vi "Configure Auto Detect.vi"(6 "Manual Frequency (0 Hz)":i32, 7 "Frequency Source (0: tsMeasFreq)":i32(ring) items=["tsMeasFreq", "tsAnlgGenA", "tsAnlgGenB", "tsDigGenA", "tsDigGenB", "tsSweepSrc0", "tsSweepSrc1"], 8 "error in (no error)":errorcluster, 9 "Enable TDD Frequency Status (0: tmFixed)":i32(ring) items=["tmFixed", "tmTuned"], 10 "Analyzer (0: A0)":i32(ring) items=["A0", "A1"], 11 "VISA resource name":refnum<visa-resource-name>) -> (0 "error out":errorcluster, 3 "VISA resource name out":refnum<visa-resource-name>)   [LabVIEW 2014, in "Stanford Research SR1.lvlib"]
doc: "Configures the attributes for the Auto Detect."
uses:
  Stanford Research SR1.lvlib
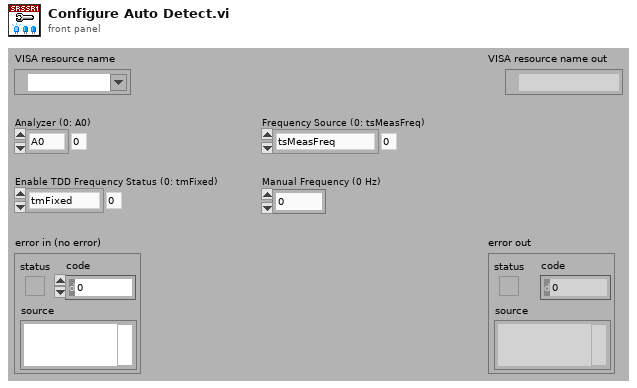
[diagram p1: front panel]
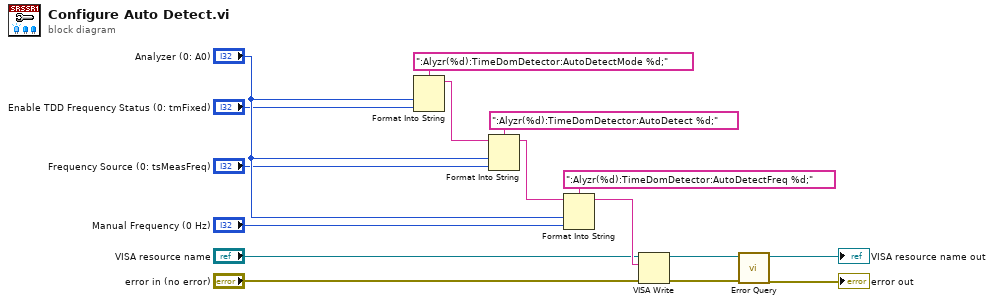
[diagram p0: block diagram]
diagram:
  n1 = Format Into String(format string=":Alyzr(%d):TimeDomDetector:AutoDetectMode %d;", "Analyzer (0: A0)", "Enable TDD Frequency Status (0: tmFixed)") -> (resulting string=w15:string)  [unwired: 2 in, 1 out]
  n2 = Format Into String(format string=":Alyzr(%d):TimeDomDetector:AutoDetect %d;", initial string=w15, "Analyzer (0: A0)", "Frequency Source (0: tsMeasFreq)") -> (resulting string=w13:string)  [unwired: 1 in, 1 out]
  n3 = Format Into String(format string=":Alyzr(%d):TimeDomDetector:AutoDetectFreq %d;", initial string=w13, "Analyzer (0: A0)", "Manual Frequency (0 Hz)") -> (resulting string=w11:string)  [unwired: 1 in, 1 out]
  n4 = VISA Write(VISA resource name="VISA resource name", write buffer=w11, error in (no error)="error in (no error)") -> (VISA resource name out=w8:refnum<visa-resource-name>, error out=w7:errorcluster)  [unwired: 1 out]
  n5 = call "Error Query.vi"("error in (no error)"=w7, "VISA resource name"=w8) -> ("error out"=→"error out":errorcluster, "VISA resource name out"=→"VISA resource name out":refnum<visa-resource-name>)  [unwired: 6 in, 2 out]
